vi "Configure Multi Eval Meas Limit Power Dynamics OFF Power.vi"(8 "error in (no error)":errorcluster, 9 "Off Power (-50)":dbl=-50.0 format="%^.3e", 10 "Instance (1)":T1=1, 11 "VISA resource name":refnum<visa-resource-name>) -> (0 "error out":errorcluster, 3 "VISA resource name out":refnum<visa-resource-name>)   [LabVIEW 2020, in "Rohde&Schwarz CMWXP NR FR1 Measurement.lvlib"]
doc: "Defines an upper limit for the OFF power determined with the power dynamics measurement.\n\nAttribute:\nRSCMWXPNRFR1M_ATTR_MULTI_EVAL_MEAS_LIMIT_POWER_DYNAMICS_OFF_POWER\n\nRemote-control command:\nCONFigure:NRSub:MEAS<i>:MEValuation:LIMit:PDYNamics:OFFPower"
uses:
  <instrlib>/Rohde&Schwarz CMWXP NR FR1 Measurement/Rohde&Schwarz CMWXP NR FR1 Measurement.lvlib
  <instrlib>/Rohde&Schwarz CMWXP NR FR1 Measurement/Private/_Instance.ctl
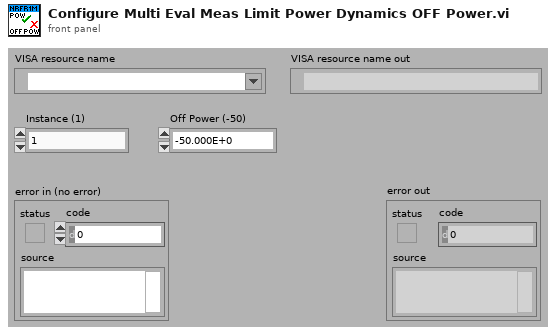
[diagram p1: front panel]
types:
  T1 = typedef "Rohde&Schwarz CMWXP NR FR1 Measurement.lvlib/_Instance.ctl" = i32
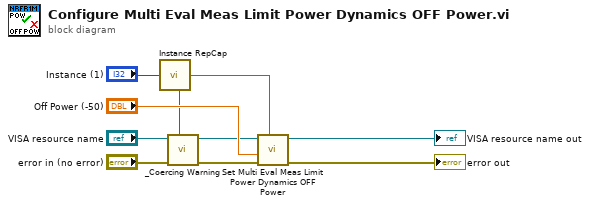
[diagram p0: block diagram]
diagram:
  n1 = call <instrlib>:"Instance RepCap.vi"("Instance In"="Instance (1)") -> ("In Range?"=w2:bool, "RepCap Identifier Out"=w6:string)  [unwired: 1 in]
  n2 = call <instrlib>:"_Coercing Warning.vi"("In Range?"=w2, "error in (no error)"="error in (no error)", "VISA resource name"="VISA resource name") -> ("error out"=w3:errorcluster, "VISA resource name out"=w1:refnum<visa-resource-name>)  [unwired: 7 in]
  n3 = call "Set Multi Eval Meas Limit Power Dynamics OFF Power"("Repeated Capabilities"=w6, "error in (no error)"=w3, "Multi Eval Meas Limit Power Dynamics OFF Power (0.0)"="Off Power (-50)", "instrument handle"=w1) -> ("error out"=→"error out":errorcluster, "instrument handle out"=→"VISA resource name out":refnum<visa-resource-name>)  [unwired: 6 in]
